vi "GetIOConfigurationStatusMerge.vi"   [LabVIEW 2017]
doc: "Reports the status of writing channel configuration data to I/O items."
uses:
  <vilib>/eio/EIOGrowableMethodNode/genericMethod/EIOGrowableMethodNode.xnode
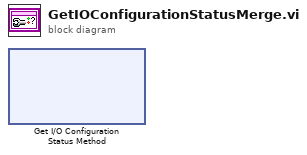
[diagram p0: block diagram]
diagram:
  n1 = xnode "Get I/O Configuration Status Method"() -> ()  [unwired: 1 in, 3 out]
